vi "Configure AC Bandwidth [AC].vi"(8 "error in (no error)":errorcluster, 9 "ac max frequency (300.0E+3 Hz)":dbl=300000.0 format="%^.2e", 10 "ac min frequency (20.0 Hz)":dbl=20.0 format="%^.2e", 11 "CS++DMM in":refnum<class "CS++DMM.lvclass">) -> (0 "error out":errorcluster, 3 "CS++DMM out":refnum<class "CS++DMM.lvclass">)   [LabVIEW 2013, in "CS++DMM.lvlib" / "CS++DMM.lvclass"]
doc: "This VI configures the AC minimum and maximum frequency for DMMs that take AC voltage or AC current measurements.\n\nThis VI affects the behavior of the instrument only if the IviDmm>Basic Operation>Function property is set to an AC voltage or AC current measurement.\n\nNote:\n\n(1) This VI is part of the IviDmmACMeasurement [AC] extension group."
uses:
  CS++DMM.lvclass
  CSPP_Core/Classes/CS++ProcessVariables/ProcessVariable/PV.lvclass
  CSPP_Core/Classes/CS++ProcessVariables/ProcessVariable/PV.lvclass/PV.ctl
  CS++DMM.lvclass/CS++DMM.ctl
  CSPP_Core/Classes/CS++ProcessVariables/PVConnection/PVConnection.lvclass
  CSPP_Core/Classes/CS++ProcessVariables/ProcessVariable/Write Data.vi
  CSPP_Core/Classes/CS++ProcessVariables/ProcessVariable/Write Timestamp.vi
  CSPP_Core/Classes/CS++ProcessVariables/ProcessVariable/Write Quality.vi
  CSPP_Core/Classes/CS++ProcessVariables/ProcessVariable/Write status.vi
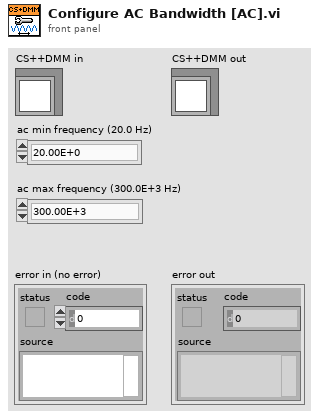
[diagram p1: front panel]
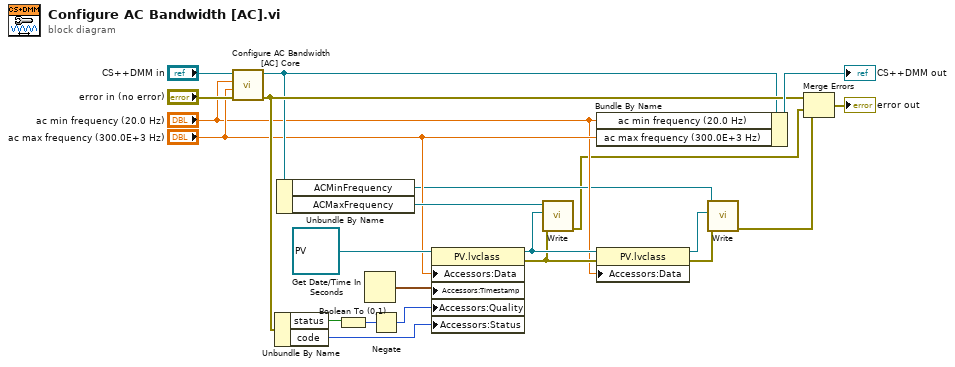
[diagram p0: block diagram]
diagram:
  n1 = call-dynamic "Configure AC Bandwidth [AC] Core.vi"("error in (no error)"="error in (no error)", "ac max frequency (300.0E+3 Hz)"="ac max frequency (300.0E+3 Hz)", "ac min frequency (20.0 Hz)"="ac min frequency (20.0 Hz)", "CS++DMM in"="CS++DMM in") -> ("error out"=w12:errorcluster, "CS++DMM out"=w11:refnum<class "CS++DMM.lvclass">)  [unwired: 6 in]
  n2 = Unbundle By Name(w12) -> ("status"=w18:bool, "code"=w15:i32)
  n3 = Unbundle By Name(w11) -> ("ACMinFrequency"=w4:refnum<class "PVConnection.lvclass">, "ACMaxFrequency"=w13:refnum<class "PVConnection.lvclass">)
  n4 = Boolean To (0,1)(Boolean=w18) -> (0, 1=w17:i16)
  n5 = Get Date/Time In Seconds() -> (seconds since 1Jan1904=w14:timestamp)
  n6 = Negate(x=w17) -> (-x=w16:i16)
  n7 = property class="PV.lvclass"(reference=refnum<class "PV.lvclass"> refnum ("CS++ProcessVariables.lvlib:PV.lvclass"), "Accessors:Data"="ac max frequency (300.0E+3 Hz)", "Accessors:Timestamp"=w14, "Accessors:Quality"=w16, "Accessors:Status"=w15) -> (reference out=w7:refnum<class "PV.lvclass">, error out=w6:errorcluster)  [unwired: 1 in]
  n8 = call-dynamic "Write.vi"("error in (no error)"=w6, "PV"=w7, "PVConnection in"=w13) -> ("error out"=w2:errorcluster)  [unwired: 7 in, 1 out]
  n9 = Bundle By Name(cluster=w11, "ac min frequency (20.0 Hz)"="ac min frequency (20.0 Hz)", "ac max frequency (300.0E+3 Hz)"="ac max frequency (300.0E+3 Hz)") -> (→"CS++DMM out":refnum<class "CS++DMM.lvclass">)
  n10 = property class="PV.lvclass"(reference=w7, error in=w6, "Accessors:Data"="ac min frequency (20.0 Hz)") -> (reference out=w9:refnum<class "PV.lvclass">, error out=w8:errorcluster)
  n11 = call-dynamic "Write.vi"("error in (no error)"=w8, "PV"=w9, "PVConnection in"=w4) -> ("error out"=w1:errorcluster)  [unwired: 7 in, 1 out]
  n12 = Merge Errors(w12, w2, w1) -> (→"error out":errorcluster)
